vi "myRIO_BRig_RT_dataExp_IallReward.vi"() -> (2 "output_I_allReward":i32)   [LabVIEW 2014]
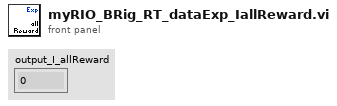
[diagram p1: front panel]
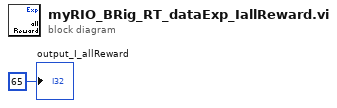
[diagram p0: block diagram]
diagram:
  "output_I_allReward" <- 65 ("output_iBlock")
